vi "Generate Data Offset.vi"(6 "Starting Address Offset":u16 format="%04x", 8 "error in (no error)":errorcluster, 11 "Remote Terminal in":refnum<class "Remote Terminal.lvclass">) -> (0 "error out":errorcluster, 3 "Remote Terminal out":refnum<class "Remote Terminal.lvclass">)   [LabVIEW 2020, in "BCI-1553 API.lvlib" / "Remote Terminal.lvclass"]
doc: "Generates the address offset for this Remote Terminal."
uses:
  Remote Terminal.lvclass
  Remote Terminal.lvclass/Remote Terminal.ctl
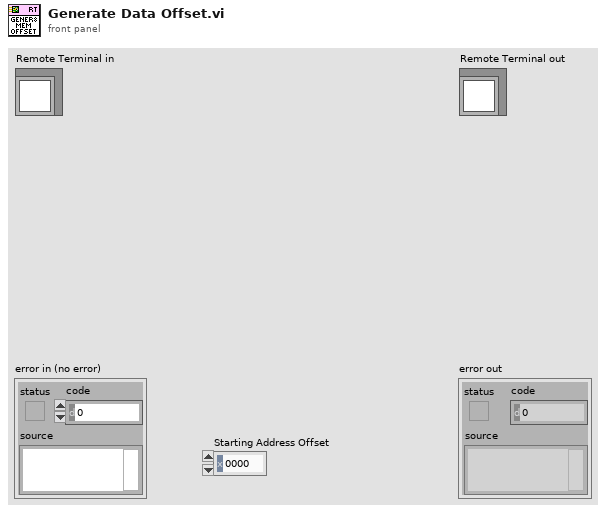
[diagram p1: front panel]
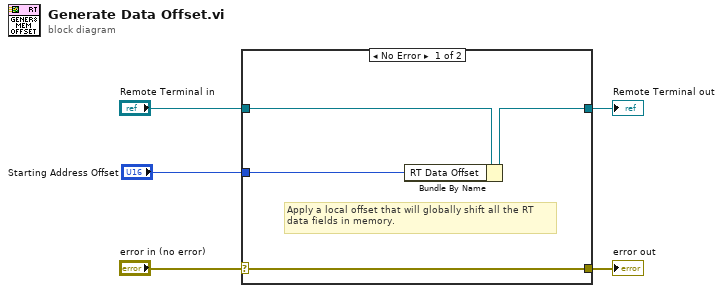
[diagram p0: block diagram]
diagram:
  n1 = case shown="No Error" "error in (no error)" {
    selector: "error in (no error)" -> [w9 w11]
    tunnel: [w9 w11] -> w4
    tunnel: [w7 w10] -> w2
    tunnel: "Remote Terminal in" -> [w8 w10]
    tunnel: "Starting Address Offset" -> [w6 _]
    frame No Error {
      # "Apply a local offset that will globally shift all the RT\ndata fields in memory."
      n2 = Bundle By Name(cluster=w8, "RT Data Offset"=w6) -> (w7:refnum<class "Remote Terminal.lvclass">)
    }
    frame Error {
    }
  }
  "error out" <- w4
  "Remote Terminal out" <- w2
